vi "FeatureStudio Body Text.vi"(4 "Input Text":string, 6 "Extrude Distance":dbl(slide) scale=0.0..10.0, 8 "Extrude?":bool, 9 "Scale":dbl(slide)=10.0 scale=0.0..1.0, 10 "rect":T1, 11 "Shape":enum16{"Text", "Rectangle", "Circle"}(ring)) -> (3 "result string":string)   [LabVIEW 2019]
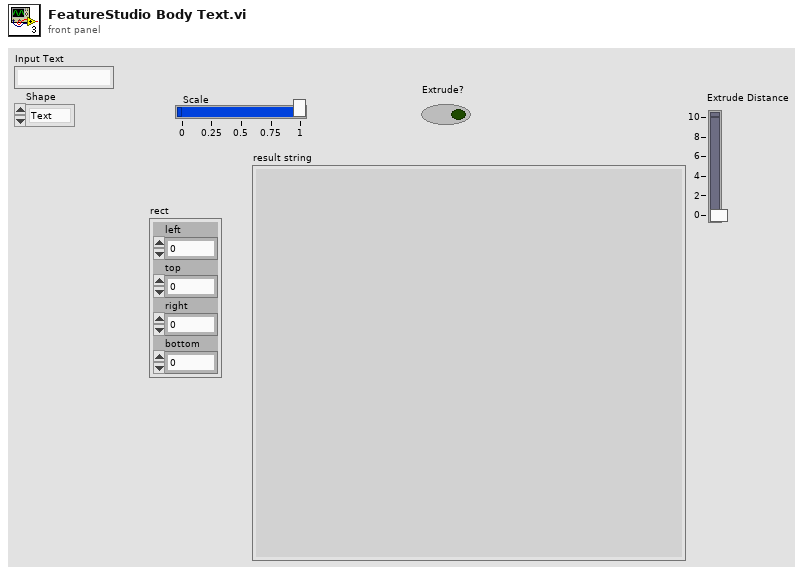
[diagram p1: front panel]
types:
  T1 = cluster{"left":i16, "top":i16, "right":i16, "bottom":i16}
  T2 = cluster{"left":dbl, "top":dbl, "right":dbl, "bottom":dbl}
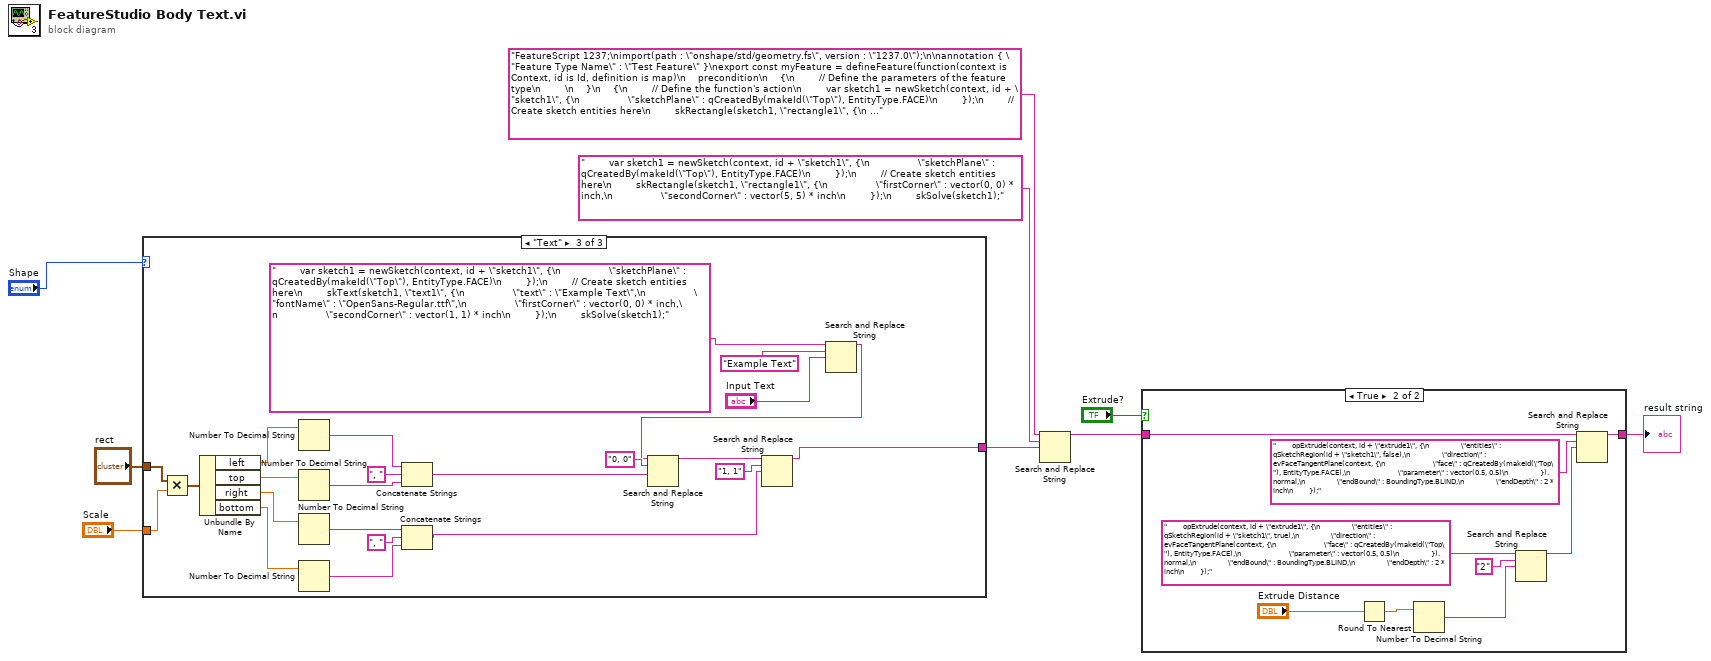
[diagram p0: block diagram]
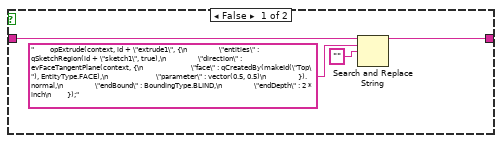
[diagram p2: hidden frame]
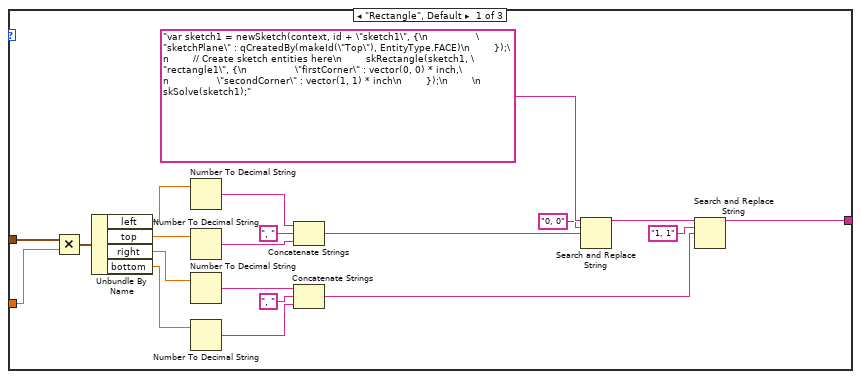
[diagram p3: hidden frame]
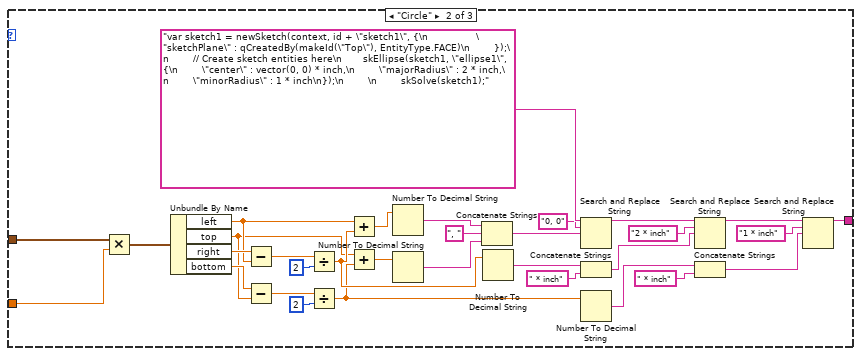
[diagram p4: hidden frame]
diagram:
  n1 = case shown="\"Text\"" "Shape" {
    tunnel: [w13 w42 w62] -> w4
    tunnel: "rect" -> [w12 w41 w73]
    tunnel: "Scale" -> [w10 w30 w72]
    frame "Rectangle", Default {
      n2 = Multiply(x=w12, y=w10) -> (x*y=w11:T2)
      n3 = Unbundle By Name(w11) -> ("left"=w29:dbl, "top"=w28:dbl, "right"=w17:dbl, "bottom"=w16:dbl)
      n4 = Number To Decimal String(number=w29) -> (decimal integer string=w25:string)  [unwired: 1 in]
      n5 = Number To Decimal String(number=w28) -> (decimal integer string=w23:string)  [unwired: 1 in]
      n6 = Number To Decimal String(number=w17) -> (decimal integer string=w14:string)  [unwired: 1 in]
      n7 = Number To Decimal String(number=w16) -> (decimal integer string=w15:string)  [unwired: 1 in]
      n8 = Concatenate Strings(w25, ", " ("regular expression"), w23) -> (w22:string)
      n9 = Concatenate Strings(w14, ", " ("regular expression"), w15) -> (w21:string)
      n10 = Search and Replace String(input string="var sketch1 = newSketch(context, id + \"sketch1\", {\n                \"sketchPlane\" : qCreatedBy(makeId(\"Top\"), EntityType.FACE)\n        });\n        // Create sketch entities here\n        skRectangle(sketch1, \"rectangle1\", {\n                \"firstCorner\" : vector(0, 0) * inch,\n                \"secondCorner\" : vector(1, 1) * inch\n        });\n        \n        skSolve(sketch1);" ("string"), search string="0, 0" ("regular expression"), replace string=w22) -> (result string=w18:string)  [unwired: 5 in, 3 out]
      n11 = Search and Replace String(input string=w18, search string="1, 1" ("regular expression"), replace string=w21) -> (result string=w13:string)  [unwired: 5 in, 3 out]
    }
    frame "Circle" {
      n12 = Multiply(x=w41, y=w30) -> (x*y=w40:T2)
      n13 = Unbundle By Name(w40) -> ("left"=w50:dbl, "top"=w31:dbl, "right"=w53:dbl, "bottom"=w32:dbl)
      n14 = Subtract(x=w53, y=w50) -> (x-y=w52:dbl)
      n15 = Subtract(x=w32, y=w31) -> (x-y=w47:dbl)
      n16 = Divide(x=w52, y=i16 2) -> (x/y=w45:dbl)
      n17 = Divide(x=w47, y=i16 2) -> (x/y=w43:dbl)
      n18 = Add(x=w50, y=w45) -> (x+y=w49:dbl)
      n19 = Add(x=w31, y=w43) -> (x+y=w46:dbl)
      n20 = Number To Decimal String(number=w49) -> (decimal integer string=w59:string)  [unwired: 1 in]
      n21 = Number To Decimal String(number=w46) -> (decimal integer string=w57:string)  [unwired: 1 in]
      n22 = Concatenate Strings(w59, ", " ("regular expression"), w57) -> (w56:string)
      n23 = Number To Decimal String(number=w45) -> (decimal integer string=w39:string)  [unwired: 1 in]
      n24 = Search and Replace String(input string="var sketch1 = newSketch(context, id + \"sketch1\", {\n                \"sketchPlane\" : qCreatedBy(makeId(\"Top\"), EntityType.FACE)\n        });\n        // Create sketch entities here\n       skEllipse(sketch1, \"ellipse1\", {\n        \"center\" : vector(0, 0) * inch,\n        \"majorRadius\" : 2 * inch,\n        \"minorRadius\" : 1 * inch\n});\n        \n        skSolve(sketch1);" ("string"), search string="0, 0" ("regular expression"), replace string=w56) -> (result string=w54:string)  [unwired: 5 in, 3 out]
      n25 = Concatenate Strings(w39, " * inch" ("regular expression")) -> (w38:string)
      n26 = Number To Decimal String(number=w43) -> (decimal integer string=w35:string)  [unwired: 1 in]
      n27 = Search and Replace String(input string=w54, search string="2 * inch" ("regular expression"), replace string=w38) -> (result string=w44:string)  [unwired: 5 in, 3 out]
      n28 = Concatenate Strings(w35, " * inch" ("regular expression")) -> (w33:string)
      n29 = Search and Replace String(input string=w44, search string="1 * inch" ("regular expression"), replace string=w33) -> (result string=w42:string)  [unwired: 5 in, 3 out]
    }
    frame "Text" {
      n30 = Multiply(x=w73, y=w72) -> (x*y=w74:T2)
      n31 = Unbundle By Name(w74) -> ("left"=w84:dbl, "top"=w83:dbl, "right"=w78:dbl, "bottom"=w77:dbl)
      n32 = Number To Decimal String(number=w84) -> (decimal integer string=w82:string)  [unwired: 1 in]
      n33 = Number To Decimal String(number=w83) -> (decimal integer string=w80:string)  [unwired: 1 in]
      n34 = Number To Decimal String(number=w78) -> (decimal integer string=w75:string)  [unwired: 1 in]
      n35 = Number To Decimal String(number=w77) -> (decimal integer string=w76:string)  [unwired: 1 in]
      n36 = Concatenate Strings(w82, ", " ("regular expression"), w80) -> (w67:string)
      n37 = Concatenate Strings(w75, ", " ("regular expression"), w76) -> (w68:string)
      n38 = Search and Replace String(input string="        var sketch1 = newSketch(context, id + \"sketch1\", {\n                \"sketchPlane\" : qCreatedBy(makeId(\"Top\"), EntityType.FACE)\n        });\n        // Create sketch entities here\n        skText(sketch1, \"text1\", {\n                \"text\" : \"Example Text\",\n                \"fontName\" : \"OpenSans-Regular.ttf\",\n                \"firstCorner\" : vector(0, 0) * inch,\n                \"secondCorner\" : vector(1, 1) * inch\n        });\n        skSolve(sketch1);" ("search string"), search string="Example Text" ("regular expression"), replace string="Input Text") -> (result string=w63:string)  [unwired: 5 in, 3 out]
      n39 = Search and Replace String(input string=w63, search string="0, 0" ("regular expression"), replace string=w67) -> (result string=w71:string)  [unwired: 5 in, 3 out]
      n40 = Search and Replace String(input string=w71, search string="1, 1" ("regular expression"), replace string=w68) -> (result string=w62:string)  [unwired: 5 in, 3 out]
    }
  }
  n41 = Search and Replace String(input string="FeatureScript 1237;\nimport(path : \"onshape/std/geometry.fs\", version : \"1237.0\");\n\nannotation { \"Feature Type Name\" : \"Test Feature\" }\nexport const myFeature = defineFeature(function(context is Context, id is Id, definition is map)\n    precondition\n    {\n        // Define the parameters of the feature type\n        \n    }\n    {\n        // Define the function's action\n        var sketch1 = newSketch(context, id + \"sketch1\", {\n                \"sketchPlane\" : qCreatedBy(makeId(\"Top\"), EntityType.FACE)\n        });\n        // Create sketch entities here\n        skRectangle(sketch1, \"rectangle1\", {\n                \"firstCorner\" : vector(0, 0) * inch,\n                \"secondCorner\" : vector(5, 5) * inch\n        });\n        skSolve(sketch1);\n                \n        opExtrude(context, id + \"extrude1\", {\n                \"entities\" : qSketchRegion(id + \"sketch1\", false),\n                \"direction\" : evFaceTangentPlane(context, {\n                        \"face\" : qCreatedBy(makeId(\"Top\"), EntityType.FACE),\n                        \"parameter\" : vector(0.5, 0.5)\n                }).normal,\n                \"endBound\" : BoundingType.BLIND,\n                \"endDepth\" : 2 * inch\n        });\n        \n    });" ("Python version"), search string="        var sketch1 = newSketch(context, id + \"sketch1\", {\n                \"sketchPlane\" : qCreatedBy(makeId(\"Top\"), EntityType.FACE)\n        });\n        // Create sketch entities here\n        skRectangle(sketch1, \"rectangle1\", {\n                \"firstCorner\" : vector(0, 0) * inch,\n                \"secondCorner\" : vector(5, 5) * inch\n        });\n        skSolve(sketch1);", replace string=w4) -> (result string=w3:string)  [unwired: 5 in, 3 out]
  n42 = case shown="True" "Extrude?" {
    tunnel: [w85 w96] -> w7
    tunnel: w3 -> [w87 w89]
    frame False {
      n43 = Search and Replace String(input string=w87, search string="        opExtrude(context, id + \"extrude1\", {\n                \"entities\" : qSketchRegion(id + \"sketch1\", true),\n                \"direction\" : evFaceTangentPlane(context, {\n                        \"face\" : qCreatedBy(makeId(\"Top\"), EntityType.FACE),\n                        \"parameter\" : vector(0.5, 0.5)\n                }).normal,\n                \"endBound\" : BoundingType.BLIND,\n                \"endDepth\" : 2 * inch\n        });", replace string="" ("replace string (\"\")")) -> (result string=w85:string)  [unwired: 5 in, 3 out]
    }
    frame True {
      n44 = Round To Nearest(number="Extrude Distance") -> (nearest integer value=w93:dbl)
      n45 = Number To Decimal String(number=w93) -> (decimal integer string=w91:string)  [unwired: 1 in]
      n46 = Search and Replace String(input string="        opExtrude(context, id + \"extrude1\", {\n                \"entities\" : qSketchRegion(id + \"sketch1\", true),\n                \"direction\" : evFaceTangentPlane(context, {\n                        \"face\" : qCreatedBy(makeId(\"Top\"), EntityType.FACE),\n                        \"parameter\" : vector(0.5, 0.5)\n                }).normal,\n                \"endBound\" : BoundingType.BLIND,\n                \"endDepth\" : 2 * inch\n        });" ("search string"), search string="2", replace string=w91) -> (result string=w90:string)  [unwired: 5 in, 3 out]
      n47 = Search and Replace String(input string=w89, search string="        opExtrude(context, id + \"extrude1\", {\n                \"entities\" : qSketchRegion(id + \"sketch1\", false),\n                \"direction\" : evFaceTangentPlane(context, {\n                        \"face\" : qCreatedBy(makeId(\"Top\"), EntityType.FACE),\n                        \"parameter\" : vector(0.5, 0.5)\n                }).normal,\n                \"endBound\" : BoundingType.BLIND,\n                \"endDepth\" : 2 * inch\n        });", replace string=w90) -> (result string=w96:string)  [unwired: 5 in, 3 out]
    }
  }
  "result string" <- w7
